vi "XY Graph Delete Plot.vi"(8 "Error In":errorcluster, 9 "Plot Index":i32, 11 "XYGraph Ref":T1) -> (0 "Error Out":errorcluster, 2 "Plot Name":string, 3 "XYGraph Ref":T1, 5 "Graph Caption (or Label)":string)   [LabVIEW 2021, in "XY Graph Add-Ons.lvlib"]
uses:
  XY Graph Add-Ons.lvlib
  XY Graph Refnum.ctl
  Plot Update Steps.ctl
  XY Graph Plot Properties.ctl
  590ba25e-86b4-4e7d-8f34-68816edeb31e.vi
  XY Graph Get Plots Metadata.vi
  XY Graph Set Plots Metadata.vi
  Graphs.lvlib
  Error/Error.lvlib
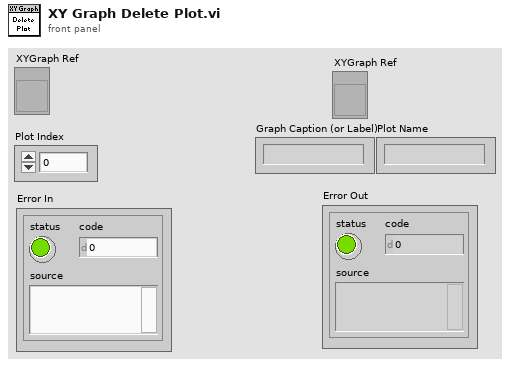
[diagram p1: front panel]
types:
  T1 = typedef "XY Graph Add-Ons.lvlib/XY Graph Refnum.ctl" = refnum<vi>
  T2 = typedef "Graphs.lvlib/Plot Update Steps.ctl" = enum16{"Update Plot Styles", "Update Annotation List", "Update Cursor List", "Update Plots", "Quit"}
  T3 = typedef "XY Graph Add-Ons.lvlib/XY Graph Plot Properties.ctl" = cluster{"PlotIndex":i32, "BarPlotStyle":u8, "DigitalLineStyle":u8, "TransitionLocation":u8, "TransitionType":u8, "FillTo":i16, "FillPointColor":u32, "LabelFormat":u8, "LineStyle":u8, "LineWidth":u8, "PlotColor":u32, "PlotInterpolation":u8, "PlotName":string, "PointStyle":u8, "Visible":bool, "XScaleIdx":u32, "YScaleIdx":u32, "AntiAliased":bool}
  T4 = typedef "LVAnnotationListTypeDef.ctl" = cluster{"Name":string, "Color":u32, "Style":u8, "Point Style":u8, "Name Visible":bool, "Allow Drag":bool, "Annotation Mode":u32, "Plot":i32, "Index":i32, "Position":cluster{"X":dbl, "Y":dbl}, "X Scale":u32, "Y Scale":u32, "Show Arrow":bool, "Lock Name":bool, "Plot Area":i32, "Label Offset":cluster{"X":dbl, "Y":dbl}}[]
  T5 = typedef "LVCursorListTypeDef.ctl" = cluster{"Name":string, "Color":u32, "Style":u8, "Point Style":u8, "Name Visible":bool, "Allow Drag":bool, "Cursor Mode":u32, "Plot":i32, "Index":i32, "Position":cluster{"X":dbl, "Y":dbl}, "X Scale":u32, "Y Scale":u32, "Watch Plots":i32[], "Watch All Plots":bool, "Plot Area":i32, "Label Offset":cluster{"X":dbl, "Y":dbl}}[]
  T6 = cluster{"Name":string, "Color":u32, "Style":u8, "Point Style":u8, "Name Visible":bool, "Allow Drag":bool, "Annotation Mode":u32, "Plot":i32, "Index":i32, "Position":cluster{"X":dbl, "Y":dbl}, "X Scale":u32, "Y Scale":u32, "Show Arrow":bool, "Lock Name":bool, "Plot Area":i32, "Label Offset":cluster{"X":dbl, "Y":dbl}}
  T7 = cluster{"Name":string, "Color":u32, "Style":u8, "Point Style":u8, "Name Visible":bool, "Allow Drag":bool, "Cursor Mode":u32, "Plot":i32, "Index":i32, "Position":cluster{"X":dbl, "Y":dbl}, "X Scale":u32, "Y Scale":u32, "Watch Plots":i32[], "Watch All Plots":bool, "Plot Area":i32, "Label Offset":cluster{"X":dbl, "Y":dbl}}
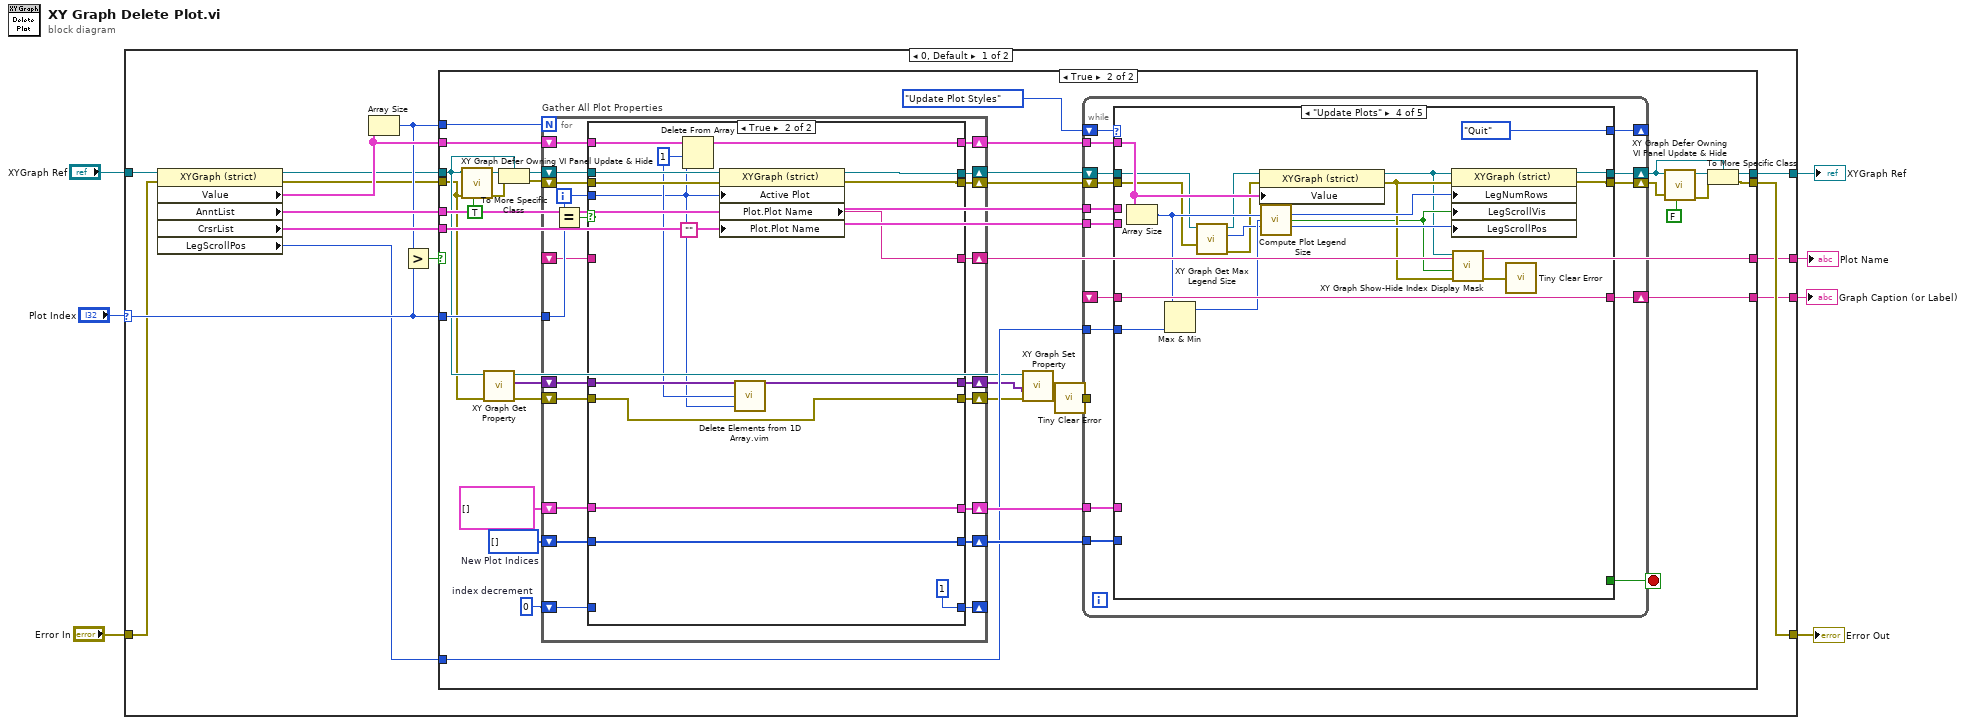
[diagram p0: block diagram]
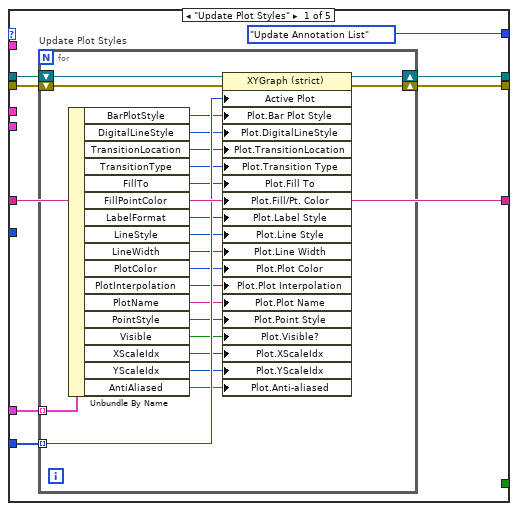
[diagram p3: hidden frame]
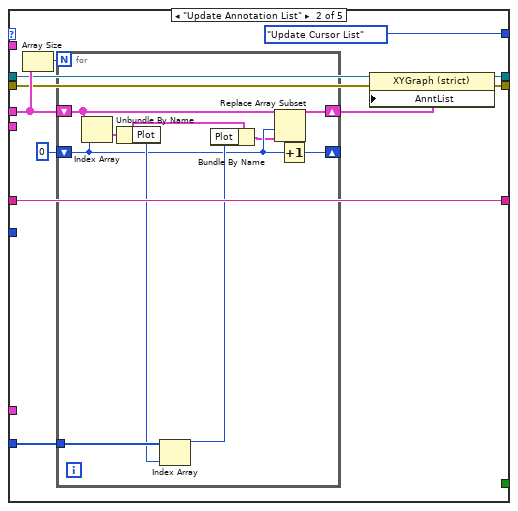
[diagram p4: hidden frame]
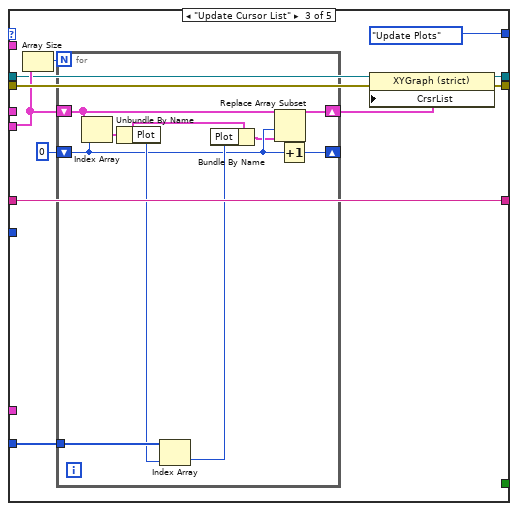
[diagram p5: hidden frame]
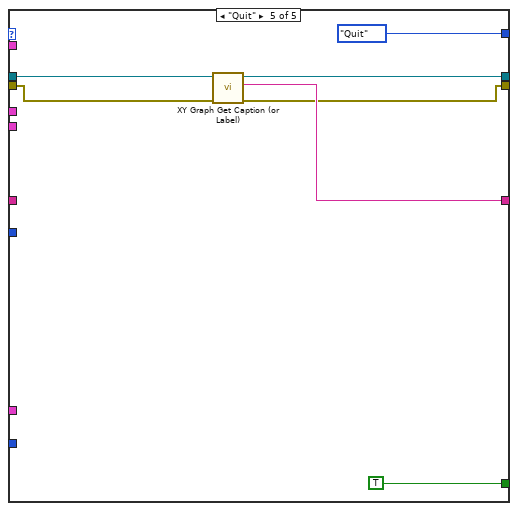
[diagram p6: hidden frame]
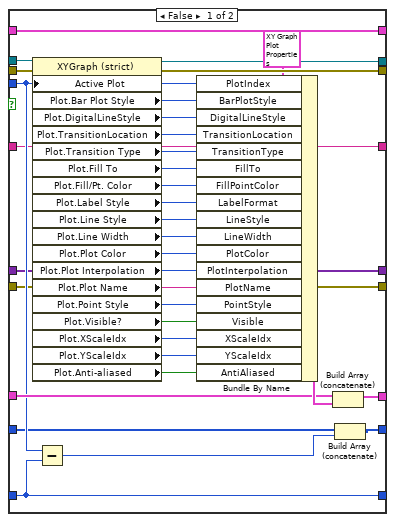
[diagram p7: hidden frame]
diagram:
  n1 = case shown="0, Default" "Plot Index" {
    selector: "Plot Index" -> [w15 _]
    tunnel: "XYGraph Ref" -> [w11 w247]
    tunnel: [w20 w247] -> w5
    tunnel: "Error In" -> [w10 w246]
    tunnel: [w19 w246] -> w3
    tunnel: [w17 _] -> w2
    tunnel: [w16 _] -> w1
    frame 0, Default {
      n2 = property class="XYGraph (strict)"(reference=w11, error in=w10) -> (reference out=w9:T1, error out=w8:errorcluster, "Value"=w22:cluster{"X Array":dbl[], "Y Array":dbl[]}[], "AnntList"=w21:T4, "CrsrList"=w18:T5, "LegScrollPos"=w12:u32)
      n3 = Array Size(array=w22) -> (size(s)=w14:i32)
      n4 = Greater?(x=w14, y=w15) -> (0:w13:bool)
      n5 = case shown="True" w13 {
        tunnel: w8 -> [w23 w32]
        tunnel: w22 -> [_ w61]
        tunnel: w21 -> [_ w55]
        tunnel: [w24 w37] -> w20
        tunnel: [w23 w34] -> w19
        tunnel: w18 -> [_ w53]
        tunnel: w9 -> [w24 w33]
        tunnel: [_ w52] -> w17
        tunnel: [_ w51] -> w16
        tunnel: w15 -> [_ w50]
        tunnel: w14 -> [_ w49]
        tunnel: w12 -> [_ w48]
        frame False {
        }
        frame True {
          w58 = i32[] []  # New Plot Indices
          w60 = 0  # index decrement
          n6 = call "XY Graph Defer Owning VI Panel Update & Hide.vi"("Defer Owning Panel Update"=TRUE, "error in (no error)"=w32, "XY Graph Refnum in"=w33) -> ("error out"=w39:errorcluster, "XY Graph Refnum out"=w41:refnum<vi>)  [unwired: 7 in]
          n7 = call-poly "XY Graph Get Property.vi"("Error In"=w32, "XYGraph Ref"=w33) -> ("Error Out"=w31:errorcluster, "Plot Metadata"=w30:variant[], "XYGraph Ref (dup)"=w26:T1)  [unwired: 6 in, 1 out]
          n8 = To More Specific Class(target class=w33, reference=w41, error in=w39) -> (specific class reference=w40:T1, error out=w38:errorcluster)
          n9 = for "Gather All Plot Properties" {
            N: w49 -> [_]
            tunnel: w50 -> [w193]
            shift-right: [w190] -> w54
            shift-left: w61 -> [w191]
            shift-right: [w185] -> w59
            shift-left: T3[] [] -> [w186]
            shift-right: [w187] -> w46
            shift-left: w38 -> [w188]
            shift-right: [w183] -> _
            shift-left: w60 -> [w184]
            shift-right: [w181] -> w57
            shift-left: w58 -> [w182]
            shift-right: [w189] -> w47
            shift-left: w40 -> [w195]
            shift-right: [w180] -> w51
            shift-left: _ -> [w179]
            shift-right: [w177] -> w29
            shift-left: w31 -> [w178]
            shift-right: [w175] -> w25
            shift-left: w30 -> [w176]
            i -> [w194]
            n10 = Equal?(x=w194, y=w193) -> (x = y?=w192:bool)
            n11 = case shown="True" w192 {
              tunnel: w195 -> [w229 w243]
              tunnel: w194 -> [w204 w232]
              tunnel: w191 -> [w228 w245]
              tunnel: [w228 w244] -> w190
              tunnel: [w227 w239] -> w189
              tunnel: w188 -> [w226 w238]
              tunnel: [w225 w237] -> w187
              tunnel: w186 -> [w206 w242]
              tunnel: [w205 w242] -> w185
              tunnel: w184 -> [w203 _]
              tunnel: [w203 1 ("index decrement")] -> w183
              tunnel: w182 -> [w202 w240]
              tunnel: [w200 w240] -> w181
              tunnel: [w199 w236] -> w180
              tunnel: w179 -> [w199 _]
              tunnel: w178 -> [w197 w230]
              tunnel: [w197 w230] -> w177
              tunnel: w176 -> [w196 w234]
              tunnel: [w196 w231] -> w175
              frame False {
                n12 = property class="XYGraph (strict)"(reference=w229, error in=w226, "Active Plot"=w204) -> (reference out=w227:T1, error out=w225:errorcluster, "Plot.Bar Plot Style"=w224:u8, "Plot.DigitalLineStyle"=w223:u8, "Plot.TransitionLocation"=w222:u8, "Plot.Transition Type"=w221:u8, "Plot.Fill To"=w220:i16, "Plot.Fill/Pt. Color"=w219:u32, "Plot.Label Style"=w218:u8, "Plot.Line Style"=w217:u8, "Plot.Line Width"=w216:u8, "Plot.Plot Color"=w215:u32, "Plot.Plot Interpolation"=w214:u8, "Plot.Plot Name"=w213:string, "Plot.Point Style"=w212:u8, "Plot.Visible?"=w211:bool, "Plot.XScaleIdx"=w210:u32, "Plot.YScaleIdx"=w209:u32, "Plot.Anti-aliased"=w198:bool)
                n13 = Subtract(x=w204, y=w203) -> (x-y=w201:i32)
                n14 = Bundle By Name(cluster=T3 {"PlotIndex"=0, "BarPlotStyle"=0, "DigitalLineStyle"=0, "TransitionLocation"=0, "TransitionType"=0, "FillTo"=0, "FillPointColor"=0, "LabelFormat"=0, "LineStyle"=0, "LineWidth"=0, "PlotColor"=0, "PlotInterpolation"=0, "PlotName"="", "PointStyle"=0, "Visible"=FALSE, "XScaleIdx"=0, "YScaleIdx"=0, "AntiAliased"=FALSE}, "PlotIndex"=w204, "BarPlotStyle"=w224, "DigitalLineStyle"=w223, "TransitionLocation"=w222, "TransitionType"=w221, "FillTo"=w220, "FillPointColor"=w219, "LabelFormat"=w218, "LineStyle"=w217, "LineWidth"=w216, "PlotColor"=w215, "PlotInterpolation"=w214, "PlotName"=w213, "PointStyle"=w212, "Visible"=w211, "XScaleIdx"=w210, "YScaleIdx"=w209, "AntiAliased"=w198) -> (w207:T3)
                n15 = Build Array (concatenate)(w206, w207) -> (w205:T3[])
                n16 = Build Array (concatenate)(w202, w201) -> (w200:i32[])
              }
              frame True {
                w233 = 1 ("length")
                n17 = Delete From Array(array=w245, length=w233, index=w232) -> (array with subset deleted=w244:cluster{"X Array":dbl[], "Y Array":dbl[]}[])  [unwired: 1 out]
                n18 = property class="XYGraph (strict)"(reference=w243, error in=w238, "Active Plot"=w232, "Plot.Plot Name"="") -> (reference out=w239:T1, error out=w237:errorcluster, "Plot.Plot Name"=w236:string)
                n19 = call "Delete Elements from 1D Array.vim"("index (last elem)"=w232, "length (1)"=w233, "Array"=w234) -> ("array w/ subset deleted"=w231:variant[])  [unwired: 1 out]
              }
            }
          }
          n20 = call-poly "XY Graph Set Property.vi"("error in (no error)"=w29, "Plots Metadata"=w25, "XY Graph Refnum"=w26) -> ("error out"=w28:errorcluster)  [unwired: 7 in, 1 out]
          n21 = call "Tiny Clear Error.vi"("Error In"=w28) -> ("no Error Out"=w27:errorcluster)  [unwired: 8 in]
          n22 = while {
            tunnel: w59 -> [w77]
            tunnel: w57 -> [w74]
            shift-right: [w71] -> _
            shift-left: Plot_Update_Steps."Update Plot Styles" -> [w73]
            shift-right: [w63] -> w43
            shift-left: w46 -> [w75]
            tunnel: w55 -> [w70]
            tunnel: w54 -> [w69]
            tunnel: w53 -> [w68]
            shift-right: [w64] -> w36
            shift-left: w47 -> [w76]
            shift-right: [w67] -> w52
            shift-left: _ -> [w66]
            tunnel: w48 -> [w65]
            tunnel: w27 -> [_]
            stop <- w72 stop-if-true
            n23 = case shown="\"Update Plots\"" w73 {
              tunnel: w77 -> [w85 _ _ _ _]
              tunnel: w76 -> [w84 w114 w129 w155 w173]
              tunnel: w75 -> [w83 w112 w134 w153 w169]
              tunnel: [w82 w111 w133 w164 w168] -> w63
              tunnel: [w81 w113 w135 w165 w170] -> w64
              tunnel: w74 -> [w80 w118 w138 _ _]
              tunnel: [_ _ _ _ TRUE] -> w72
              tunnel: [Plot_Update_Steps."Update Annotation List" Plot_Update_Steps."Update Cursor List" Plot_Update_Steps."Update Plots" Plot_Update_Steps."Quit" Plot_Update_Steps."Quit"] -> w71
              tunnel: w70 -> [_ w117 _ _ _]
              tunnel: w69 -> [_ _ _ w166 _]
              tunnel: w68 -> [_ _ w131 _ _]
              tunnel: [w78 w109 w130 w163 w171] -> w67
              tunnel: w66 -> [w78 w109 w130 w163 _]
              tunnel: w65 -> [_ _ _ w161 _]
              frame "Update Plot Styles" {
                n24 = for "Update Plot Styles" {
                  tunnel: w85 -> [w108] mode=indexing
                  shift-right: [w104] -> w82
                  shift-left: w83 -> [w105]
                  tunnel: w80 -> [w103] mode=indexing
                  shift-right: [w106] -> w81
                  shift-left: w84 -> [w107]
                  n25 = Unbundle By Name(w108) -> ("BarPlotStyle"=w102:u8, "DigitalLineStyle"=w101:u8, "TransitionLocation"=w100:u8, "TransitionType"=w99:u8, "FillTo"=w98:i16, "FillPointColor"=w97:u32, "LabelFormat"=w96:u8, "LineStyle"=w95:u8, "LineWidth"=w94:u8, "PlotColor"=w93:u32, "PlotInterpolation"=w92:u8, "PlotName"=w91:string, "PointStyle"=w90:u8, "Visible"=w89:bool, "XScaleIdx"=w88:u32, "YScaleIdx"=w87:u32, "AntiAliased"=w86:bool)
                  n26 = property class="XYGraph (strict)"(reference=w107, error in=w105, "Active Plot"=w103, "Plot.Bar Plot Style"=w102, "Plot.DigitalLineStyle"=w101, "Plot.TransitionLocation"=w100, "Plot.Transition Type"=w99, "Plot.Fill To"=w98, "Plot.Fill/Pt. Color"=w97, "Plot.Label Style"=w96, "Plot.Line Style"=w95, "Plot.Line Width"=w94, "Plot.Plot Color"=w93, "Plot.Plot Interpolation"=w92, "Plot.Plot Name"=w91, "Plot.Point Style"=w90, "Plot.Visible?"=w89, "Plot.XScaleIdx"=w88, "Plot.YScaleIdx"=w87, "Plot.Anti-aliased"=w86) -> (reference out=w106:T1, error out=w104:errorcluster)
                }
              }
              frame "Update Annotation List" {
                n27 = Array Size(array=w117) -> (size(s)=w116:i32)
                n28 = for {
                  N: w116 -> [_]
                  tunnel: w118 -> [w128]
                  shift-right: [w122] -> w110
                  shift-left: w117 -> [w124]
                  shift-right: [w121] -> _
                  shift-left: 0 -> [w123]
                  n29 = Index Array(array=w124, index=w123) -> (element=w126:T6)
                  n30 = Unbundle By Name(w126) -> ("Plot"=w127:i32)
                  n31 = Index Array(array=w128, index=w127) -> (element=w125:i32)
                  n32 = Bundle By Name(cluster=w126, "Plot"=w125) -> (w120:T6)
                  n33 = Replace Array Subset(array=w124, new element=w120, index=w123) -> (w122:T4)
                  n34 = Increment(x=w123) -> (x+1=w121:i32)
                }
                n35 = property class="XYGraph (strict)"(reference=w114, error in=w112, "AnntList"=w110) -> (reference out=w113:T1, error out=w111:errorcluster)
              }
              frame "Update Cursor List" {
                n36 = Array Size(array=w131) -> (size(s)=w137:i32)
                n37 = for {
                  N: w137 -> [_]
                  tunnel: w138 -> [w148]
                  shift-right: [w142] -> w132
                  shift-left: w131 -> [w144]
                  shift-right: [w141] -> _
                  shift-left: 0 -> [w143]
                  n38 = Index Array(array=w144, index=w143) -> (element=w146:T7)
                  n39 = Unbundle By Name(w146) -> ("Plot"=w147:i32)
                  n40 = Index Array(array=w148, index=w147) -> (element=w145:i32)
                  n41 = Bundle By Name(cluster=w146, "Plot"=w145) -> (w140:T7)
                  n42 = Replace Array Subset(array=w144, new element=w140, index=w143) -> (w142:T5)
                  n43 = Increment(x=w143) -> (x+1=w141:i32)
                }
                n44 = property class="XYGraph (strict)"(reference=w129, error in=w134, "CrsrList"=w132) -> (reference out=w135:T1, error out=w133:errorcluster)
              }
              frame "Update Plots" {
                n45 = Array Size(array=w166) -> (size(s)=w160:i32)
                n46 = Max & Min(x=w160, y=w161) -> (max(x,y)=w162:u32)  [unwired: 1 out]
                n47 = call "XY Graph Get Max Legend Size.vi"("Error In"=w153, "XYGraph Refnum"=w155) -> ("Error Out"=w154:errorcluster, "Max Legend Size"=w157:i32, "XYGraph Refnum"=w156:T1)  [unwired: 6 in, 1 out]
                n48 = property class="XYGraph (strict)"(reference=w156, error in=w154, "Value"=w166) -> (reference out=w150:T1, error out=w152:errorcluster)
                n49 = call "Compute Plot Legend Size.vi"("# Plots"=w160, "Current Plot (Last)"=w162, "Max Legend Size"=w157) -> ("LegNumRows"=w159:u32, "LegScrollVis"=w151:bool, "LegScrollPos"=w158:u32)  [unwired: 10 in]
                n50 = property class="XYGraph (strict)"(reference=w150, error in=w152, "LegNumRows"=w159, "LegScrollVis"=w151, "LegScrollPos"=w158) -> (reference out=w165:T1, error out=w164:errorcluster)
                n51 = call "XY Graph Show-Hide Index Display Mask.vi"("error in (no error)"=w152, "Show(T)/Hide(F)"=w151, "XYGraph Ref"=w150) -> ("error out"=w149:errorcluster)  [unwired: 7 in, 1 out]
                n52 = call "Tiny Clear Error.vi"("Error In"=w149) -> ()  [unwired: 8 in, 1 out]
              }
              frame "Quit" {
                n53 = call "XY Graph Get Caption (or Label).vi"("error in (no error)"=w169, "XY Graph in"=w173) -> ("error out"=w168:errorcluster, "Caption (or Label) Text"=w171:string, "XY Graph out"=w170:T1)  [unwired: 7 in]
              }
            }
          }
          n54 = call "XY Graph Defer Owning VI Panel Update & Hide.vi"("Defer Owning Panel Update"=FALSE, "error in (no error)"=w43, "XY Graph Refnum in"=w36) -> ("error out"=w35:errorcluster, "XY Graph Refnum out"=w44:refnum<vi>)  [unwired: 7 in]
          n55 = To More Specific Class(target class=w36, reference=w44, error in=w35) -> (specific class reference=w37:T1, error out=w34:errorcluster)
        }
      }
    }
    frame ..-1 {
    }
  }
  "XYGraph Ref" <- w5
  "Error Out" <- w3
  "Graph Caption (or Label)" <- w2
  "Plot Name" <- w1
